vi "AlliGator Phasor Calibration Map Series Dialog.vi"(5 "error in (no error)":errorcluster) -> (14 "File Name (# Steps will be added)":string, 15 "Destination Folder":path, 16 "Gate Step Series":string, 17 "Phasor Calibration Dataset Path":path, 18 "OK":bool, 19 "error out":errorcluster)   [LabVIEW 2021, in "AlliGator Scripts.lvlib"]
doc: "Dialog to enter the parameters necessary for the calculation of a Series of Phasor Calibration Maps differing by the gate step used when loading the FLI dataset."
uses:
  AlliGator Scripts.lvlib
panel:
  in  "File Name (# Steps will be added)":string
  in  "Destination Folder":path
  in  "Gate Step Series":string
  in  "Phasor Calibration Dataset Path":path
  in  "Cancel":bool
  in  "OK2":bool
  # "Enter the following information to compute the series\nof Phasor Calibration Maps:"
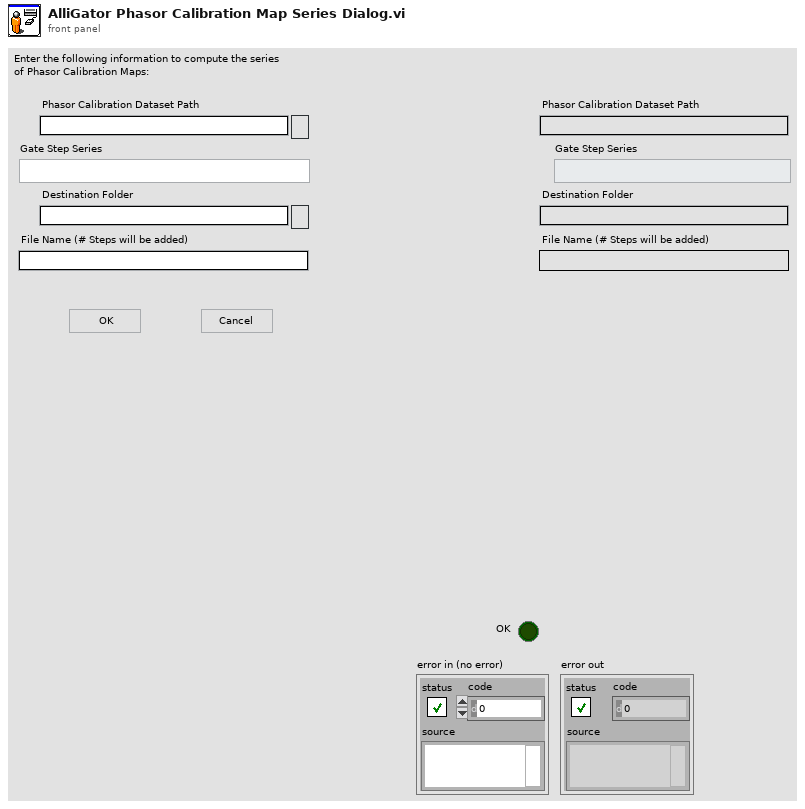
[diagram p1: front panel]
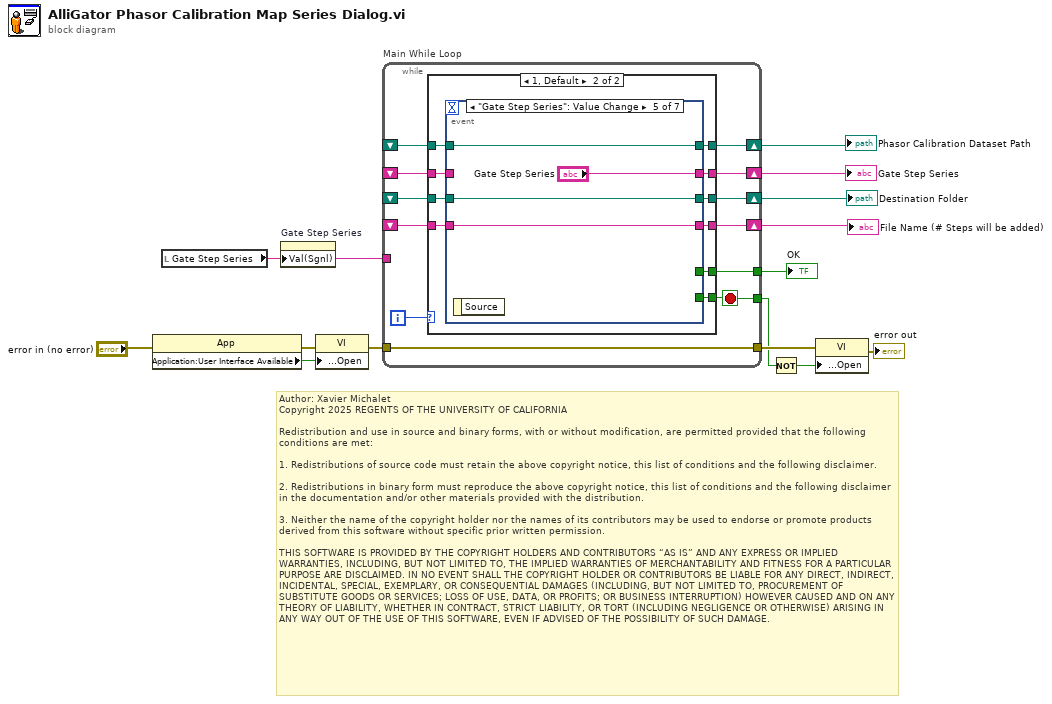
[diagram p0: block diagram]
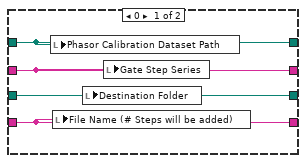
[diagram p2: hidden frame]
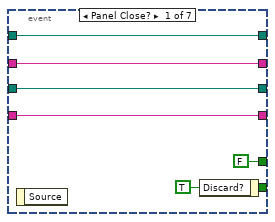
[diagram p3: hidden frame]
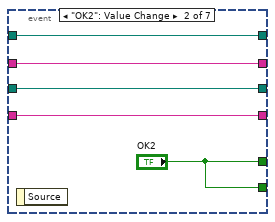
[diagram p4: hidden frame]
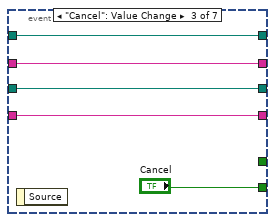
[diagram p5: hidden frame]
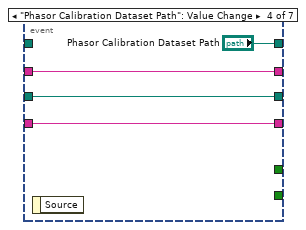
[diagram p6: hidden frame]
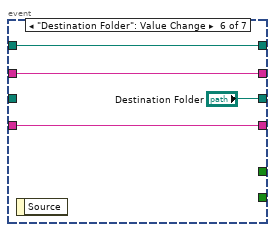
[diagram p7: hidden frame]
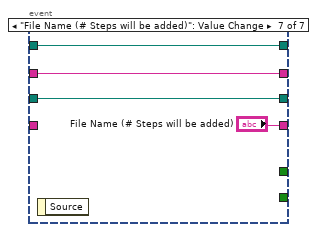
[diagram p8: hidden frame]
diagram:
  # "Author: Xavier Michalet\nCopyright 2025 REGENTS OF THE UNIVERSITY OF CALIFORNIA\n\nRedistribution and use in source and binary forms, with or without modification, are permitted provided that the following conditions are met:\n\n1. Redistributions of source code must retain the above copyright notice, this list of conditions and the following disclaimer.\n\n2. Redistributions in binary form must reproduce the above copyright notice, this list of conditions and the following disclaimer in the documentation and/or other materials provided with the distribution.\n\n3. Neither the name of the copyright holder nor the names of its contributors may be used to endorse or promote products derived from this software without specific prior written permission.\n\nTHIS SOFTWARE IS PROVIDED BY THE COPYRIGHT HOLDERS AND CONTRIBUTORS “AS IS” AND ANY EXPRESS OR IMPLIED WARRANTIES, INCLUDING, BUT NOT LIMITED TO, THE IMPLIED WARRANTIES OF MERCHANTABILITY AND FITNESS FOR A PARTICULAR PURPOSE ARE DISCLAIMED. IN NO EVENT SHALL THE COPYRIGHT HOLDER OR CONTRIBUTORS BE LIABLE FOR ANY DIRECT, INDIRECT, INCIDENTAL, SPECIAL, EXEMPLARY, OR CONSEQUENTIAL DAMAGES (INCLUDING, BUT NOT LIMITED TO, PROCUREMENT OF SUBSTITUTE GOODS OR SERVICES; LOSS OF USE, DATA, OR PROFITS; OR BUSINESS INTERRUPTION) HOWEVER CAUSED AND ON ANY THEORY OF LIABILITY, WHETHER IN CONTRACT, STRICT LIABILITY, OR TORT (INCLUDING NEGLIGENCE OR OTHERWISE) ARISING IN ANY WAY OUT OF THE USE OF THIS SOFTWARE, EVEN IF ADVISED OF THE POSSIBILITY OF SUCH DAMAGE."
  n1 = property class="App"(error in="error in (no error)") -> (error out=w9:errorcluster, "Application:User Interface Available"=w11:bool)  [unwired: 1 in, 1 out]
  n2 = local read "Gate Step Series"() -> (w1:string)
  n3 = property on="Gate Step Series" class="Str"("Val(Sgnl)"=w1) -> ()  [unwired: 2 in, 2 out]
  n4 = property class="VI"(error in=w9, "Front Panel Window:Open"=w11) -> (error out=w14:errorcluster)  [unwired: 1 in, 1 out]
  n5 = while "Main While Loop" {
    tunnel: w14 -> [w26]
    tunnel: [w26] -> w13
    tunnel: [w25] -> w8
    tunnel: [w24] -> w7
    shift-right: [w23] -> w5
    shift-left: _ -> [w21]
    shift-right: [w22] -> w4
    shift-left: _ -> [w19]
    shift-right: [w20] -> w3
    shift-left: _ -> [w17]
    shift-right: [w18] -> w2
    shift-left: _ -> [w16]
    tunnel: w1 -> [_]
    i -> [w15]
    stop <- w24 stop-if-true
    n6 = case shown="1, Default" w15 {
      tunnel: [_ w40] -> w25
      tunnel: [_ w39] -> w24
      tunnel: [w29 w38] -> w23
      tunnel: [w30 w37] -> w22
      tunnel: w21 -> [w29 w36]
      tunnel: [w27 w35] -> w20
      tunnel: w19 -> [w30 w34]
      tunnel: [w28 w33] -> w18
      tunnel: w17 -> [w27 w32]
      tunnel: w16 -> [w28 w31]
      frame 0 {
        n7 = local write "Phasor Calibration Dataset Path"(w29) -> ()
        n8 = local write "File Name (# Steps will be added)"(w28) -> ()
        n9 = local write "Destination Folder"(w27) -> ()
        n10 = local write "Gate Step Series"(w30) -> ()
      }
      frame 1, Default {
        n11 = event shown="[4] \"Gate Step Series\": Value Change" {
          selector: _ -> [_ _ _ _ _ _ _]
          dyn-events: _ -> [_ _ _ _ _ _ _]
          timeout: _ -> [_ _ _ _ _ _ _]
          tunnel: [w46 "OK2" "Cancel" _ _ _ _] -> w39
          tunnel: [FALSE ("OK") "OK2" _ _ _ _ _] -> w40
          tunnel: [w44 w50 w55 "Phasor Calibration Dataset Path" w63 w68 w72] -> w38
          tunnel: [w43 w49 w54 w59 "Gate Step Series" w66 w71] -> w37
          tunnel: w36 -> [w44 w50 w55 _ w63 w68 w72]
          tunnel: [w42 w48 w53 w58 w62 "Destination Folder" w69] -> w35
          tunnel: w34 -> [w43 w49 w54 w59 _ w66 w71]
          tunnel: [w41 w47 w52 w57 w61 w65 "File Name (# Steps will be added)"] -> w33
          tunnel: w32 -> [w42 w48 w53 w58 w62 _ w69]
          tunnel: w31 -> [w41 w47 w52 w57 w61 w65 _]
          event Panel Close? {
            w46 = TRUE ("Discard?")
            n12 = event-data() -> ()  [unwired: 1 in, 1 out]
            n13 = event-data("Discard?"=w46) -> ()  [unwired: 1 in, 1 out]
          }
          event "OK2": Value Change {
            n14 = event-data() -> ()  [unwired: 1 in, 1 out]
          }
          event "Cancel": Value Change {
            n15 = event-data() -> ()  [unwired: 1 in, 1 out]
          }
          event "Phasor Calibration Dataset Path": Value Change {
            n16 = event-data() -> ()  [unwired: 1 in, 1 out]
          }
          event "Gate Step Series": Value Change {
            n17 = event-data() -> ()  [unwired: 1 in, 1 out]
          }
          event "Destination Folder": Value Change {
            n18 = event-data() -> ()  [unwired: 1 in, 1 out]
          }
          event "File Name (# Steps will be added)": Value Change {
            n19 = event-data() -> ()  [unwired: 1 in, 1 out]
          }
        }
      }
    }
  }
  "OK" <- w8
  "Phasor Calibration Dataset Path" <- w5
  "Gate Step Series" <- w4
  "Destination Folder" <- w3
  "File Name (# Steps will be added)" <- w2
  n20 = Not(x=w7) -> (.not. x?=w6:bool)
  n21 = property class="VI"(error in=w13, "Front Panel Window:Open"=w6) -> (error out=→"error out":errorcluster)  [unwired: 1 in, 1 out]
